vi "Z-Controller Control.vi"(0 "Maximum Current":dbl=1e-08 format="%#_6p", 1 "Current Slew Rate (amps/second)":dbl=1e-10 format="%#_6p", 2 "Current Set Point":dbl=1e-10 format="%#_6p") -> ()   [LabVIEW 2017]
uses:
  <userlib>/Nanonis Prog Interface/Nanonis Prog Interface.lvlib
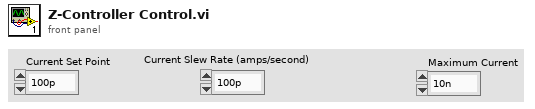
[diagram p1: front panel]
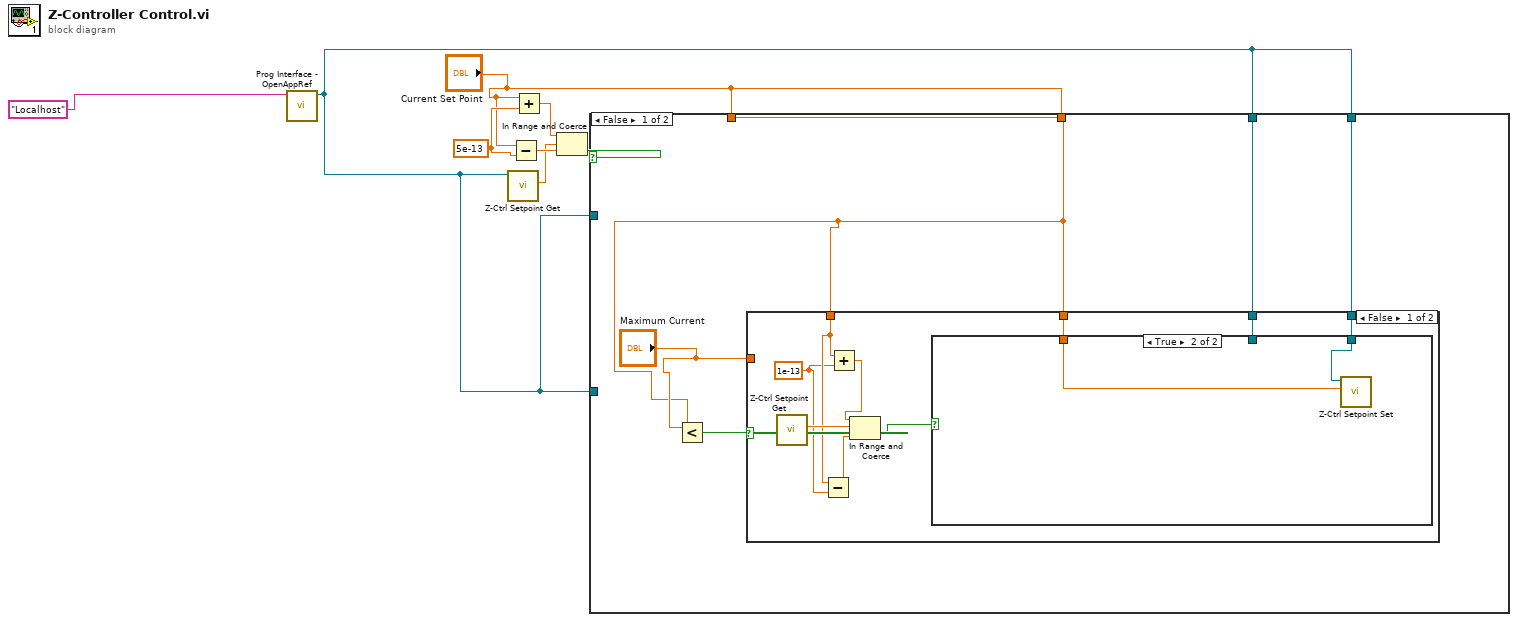
[diagram p0: block diagram]
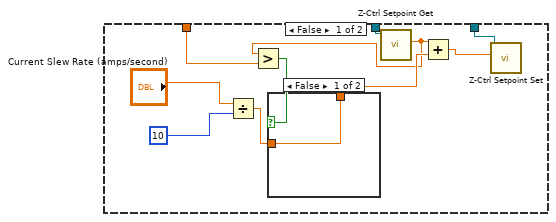
[diagram p2: hidden frame]
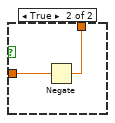
[diagram p3: hidden frame]
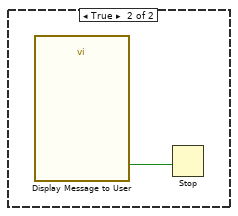
[diagram p4: hidden frame]
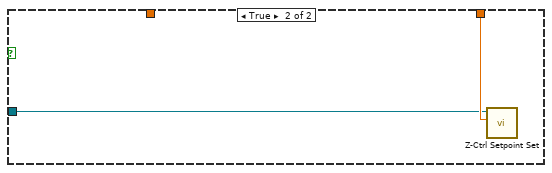
[diagram p5: hidden frame]
diagram:
  w4 = 5e-13
  n1 = call <userlib>:"Prog Interface - OpenAppRef.vi"("Machine name (local machine IP)"="Localhost") -> ("Application reference"=w1:refnum<vi>)  [unwired: 5 in, 1 out]
  n2 = call <userlib>:"Z-Ctrl Setpoint Get.vi"("Application ref in"=w1) -> ("Z Controller setpoint"=w5:sgl)  [unwired: 7 in, 2 out]
  n3 = Subtract(x="Current Set Point", y=w4) -> (x-y=w7:dbl)
  n4 = Add(x="Current Set Point", y=w4) -> (x+y=w6:dbl)
  n5 = In Range and Coerce(upper limit=w6, x=w5, lower limit=w7) -> (In Range?=w3:bool)  [unwired: 1 out]
  n6 = case shown="False" w3 {
    tunnel: "Current Set Point" -> [_ w40]
    tunnel: "Current Set Point" -> [w11 _]
    tunnel: w1 -> [_ _]
    tunnel: w1 -> [_ w39]
    tunnel: w1 -> [w10 _]
    tunnel: w1 -> [w9 _]
    frame False {
      n7 = Less?(x="Maximum Current", y=w11) -> (x < y?=w13:bool)
      n8 = case shown="False" w13 {
        tunnel: w11 -> [w22 _]
        tunnel: "Maximum Current" -> [_ _]
        tunnel: w11 -> [w20 _]
        tunnel: w10 -> [w15 _]
        tunnel: w9 -> [w14 _]
        frame False {
          w19 = 1e-13
          n9 = call <userlib>:"Z-Ctrl Setpoint Get.vi"() -> ("Z Controller setpoint"=w21:sgl)  [unwired: 8 in, 2 out]
          n10 = Subtract(x=w20, y=w19) -> (x-y=w18:dbl)
          n11 = Add(x=w20, y=w19) -> (x+y=w17:dbl)
          n12 = In Range and Coerce(upper limit=w17, x=w21, lower limit=w18) -> (In Range?=w16:bool)  [unwired: 1 out]
          n13 = case shown="True" w16 {
            tunnel: w22 -> [w31 w36]
            tunnel: w15 -> [w27 w37]
            tunnel: w14 -> [w26 _]
            frame False {
              n14 = Divide(x="Current Slew Rate (amps/second)", y=10) -> (x/y=w29:dbl)
              n15 = call <userlib>:"Z-Ctrl Setpoint Get.vi"("Application ref in"=w26) -> ("Z Controller setpoint"=w23:sgl)  [unwired: 7 in, 2 out]
              n16 = Greater?(x=w23, y=w31) -> (0:w30:bool)
              n17 = case shown="False" w30 {
                tunnel: w29 -> [w33 w35]
                tunnel: [w33 w34] -> w25
                frame False {
                }
                frame True {
                  n18 = Negate(x=w35) -> (-x=w34:dbl)
                }
              }
              n19 = Add(x=w23, y=w25) -> (x+y=w24:dbl)
              n20 = call <userlib>:"Z-Ctrl Setpoint Set.vi"("Z Controller setpoint"=w24, "Application ref in"=w27) -> ()  [unwired: 8 in, 2 out]
            }
            frame True {
              n21 = call <userlib>:"Z-Ctrl Setpoint Set.vi"("Z Controller setpoint"=w36, "Application ref in"=w37) -> ()  [unwired: 8 in, 2 out]
            }
          }
        }
        frame True {
          n22 = call "Display Message to User"() -> ("OK"=w38:bool)  [unwired: 10 in, 1 out]
          n23 = Stop(stop? (T)=w38) -> ()
        }
      }
    }
    frame True {
      n24 = call <userlib>:"Z-Ctrl Setpoint Set.vi"("Z Controller setpoint"=w40, "Application ref in"=w39) -> ()  [unwired: 8 in, 2 out]
    }
  }
